vi "Scan User ID.vi"() -> (1 "User ID Out":string, 2 "OK?":bool)   [LabVIEW 2024, in "LVarex.lvlib"]
uses:
  LVarex.lvlib
panel:
  out "In Range?":bool
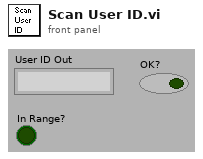
[diagram p1: front panel]
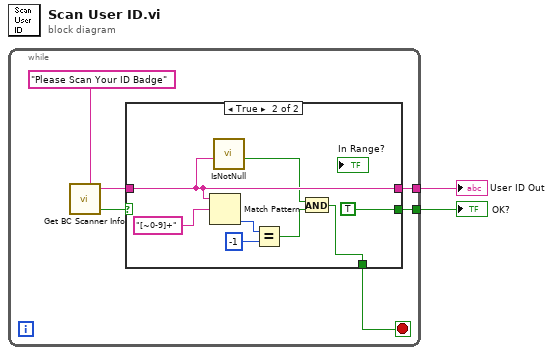
[diagram p0: block diagram]
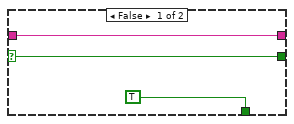
[diagram p2: hidden frame]
diagram:
  n1 = while {
    tunnel: [w4] -> w1
    tunnel: [w5] -> w2
    stop <- w3 stop-if-true
    n2 = call "Get BC Scanner Info.vi"("Prompt"="Please Scan Your ID Badge") -> ("Info Out"=w7:string, "OK"=w6:bool)  [unwired: 2 in]
    n3 = case shown="True" w6 {
      selector: w6 -> [w10 _]
      tunnel: w7 -> [w11 w13]
      tunnel: [w11 w13] -> w5
      tunnel: [w10 TRUE] -> w4
      tunnel: [TRUE w14] -> w3
      frame False {
      }
      frame True {
        n4 = Match Pattern(string=w13, regular expression="[~0-9]+") -> (offset past match=w17:i32)  [unwired: 1 in, 3 out]
        n5 = call "IsNotNull.vi"("String In"=w13) -> ("Boolean Out"=w12:bool)  [unwired: 10 in]
        n6 = Equal?(x=w17, y=-1) -> (x = y?=w15:bool)
        n7 = And(x=w12, y=w15) -> (x .and. y?=w14:bool)
      }
    }
  }
  "User ID Out" <- w2
  "OK?" <- w1
